vi "test_FPGAWrapper_FrameScan.vi"() -> ()   [LabVIEW 2010, in "FPGAWrapperMH120124FrameScan_PXI7813R.lvclass"]
uses:
  FPGAWrapperMH120124FrameScan_PXI7813R.lvclass
  common_typedefs/channels_cluster.ctl
  common/classes/ErrorController/ErrorController/ErrorController.lvclass
  common/classes/ErrorController/ErrorController/class_data.vi
panel:
  in  "zoom":dbl(slide)=1.0 scale=1.0..20.0
  in  "resolution":i32=256
  in  "amplitude in":dbl=3400.0
  out "FPGAWrapperMH120124FrameScan":refnum<class "FPGAWrapperMH120124FrameScan_PXI7813R.lvclass">
  out "error controller loaded?":bool=TRUE
  in  "number of channels":i32=3
  in  "block size":i32=10000
  out "channel data block":dbl[][](graph)
  in  "timeout (ms)":i32=500
  out "timed out?":bool
  out "samples read":i32
  out "DAQ loop counter":i32
  in  "iterations per pixel":i32=250
  out "pixel dwell time":dbl[unit]
  in  "channel offsets":T1
  in  "number of pixels":i32=1000000000
  in  "run button":bool
  in  "create button":bool
  in  "stop":bool
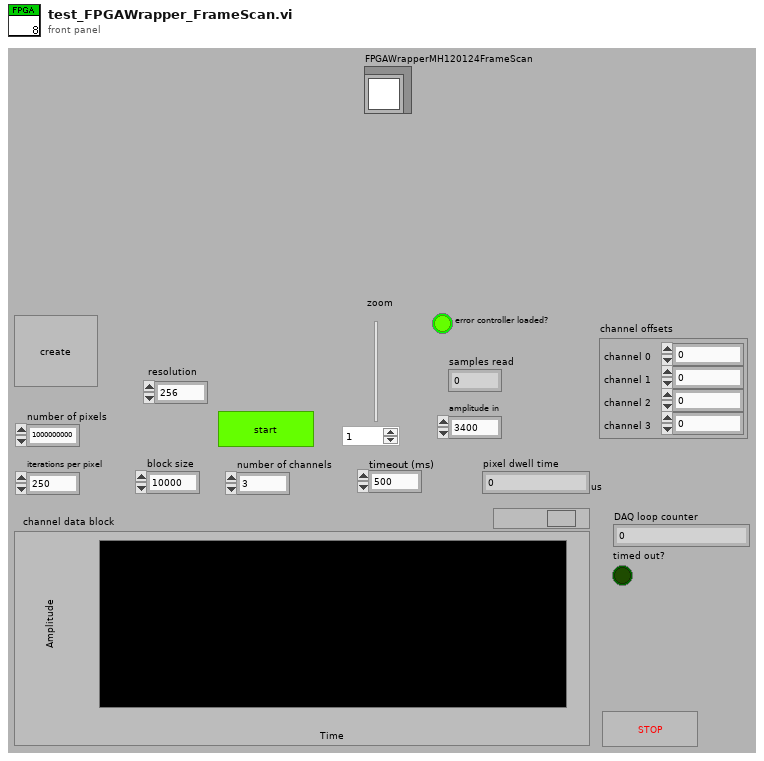
[diagram p1: front panel]
types:
  T1 = typedef "channels_cluster.ctl" = cluster{"channel 0":u32, "channel 1":u32, "channel 2":u32, "channel 3":u32}
  T2 = typedef "plugin_specification.ctl" = cluster{"class path":string, "configuration":string, "label":string, "settings name":string}
  T3 = typedef "XComponentSpecification.xctl/data.ctl" = cluster{"class path":string, "configuration":string, "label":string, "settings name":string}
  T4 = typedef "pixel_raw_data_array.ctl" = dbl[][]
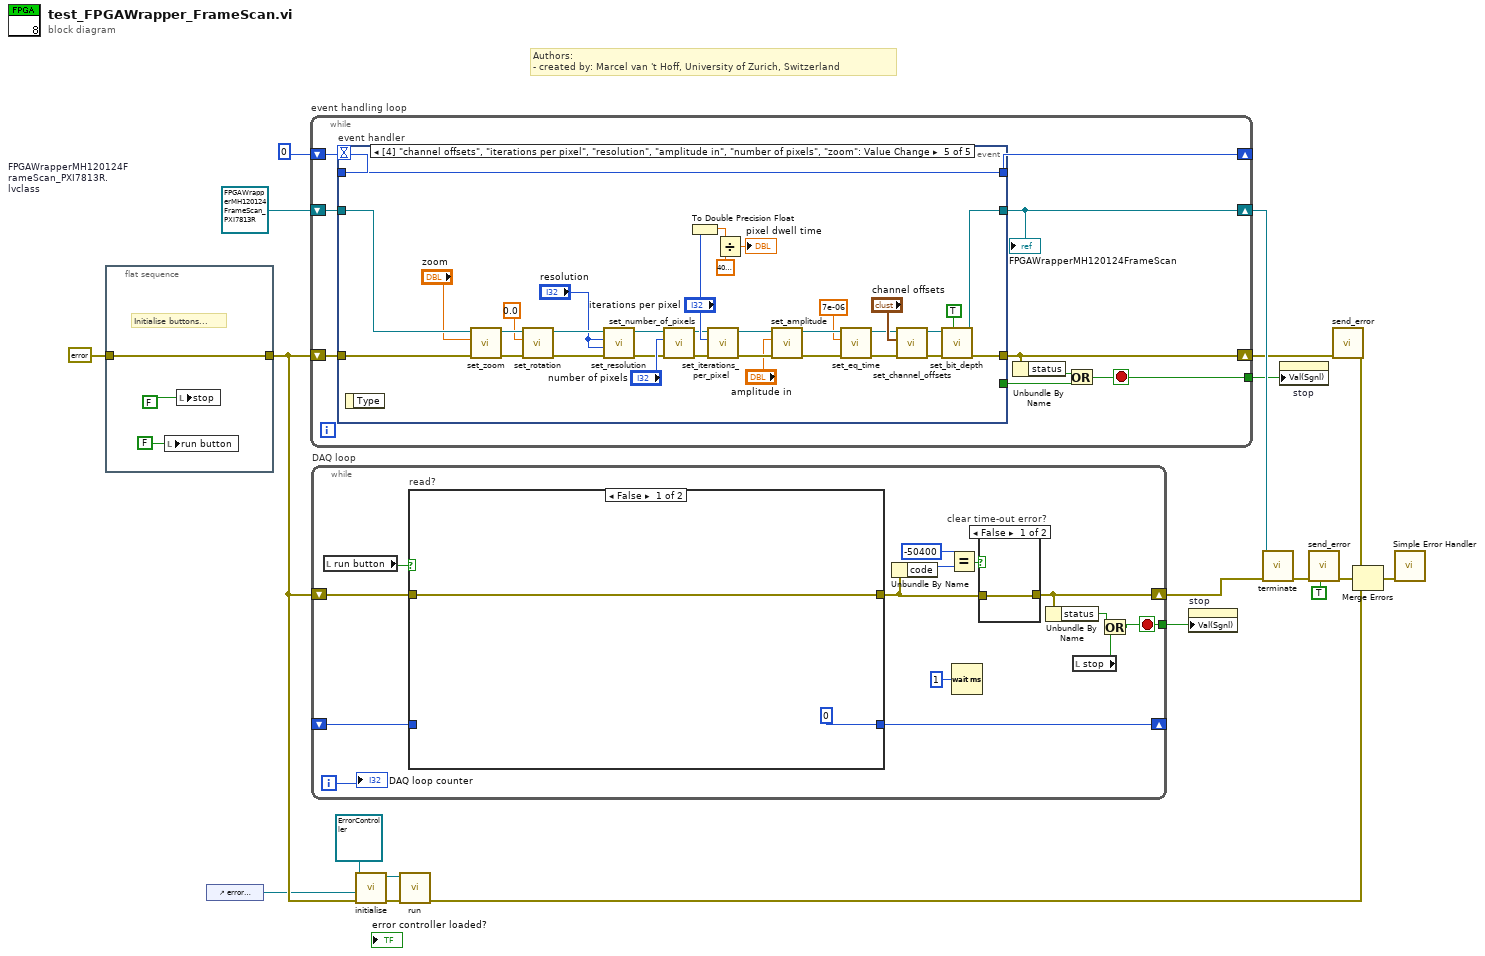
[diagram p0: block diagram]
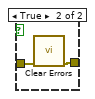
[diagram p2: hidden frame]
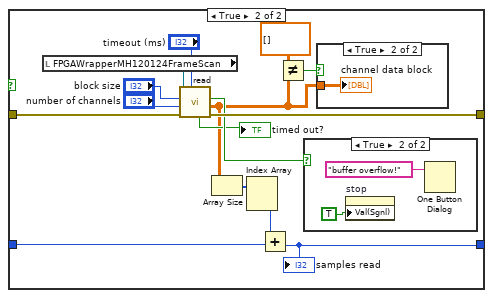
[diagram p3: hidden frame]
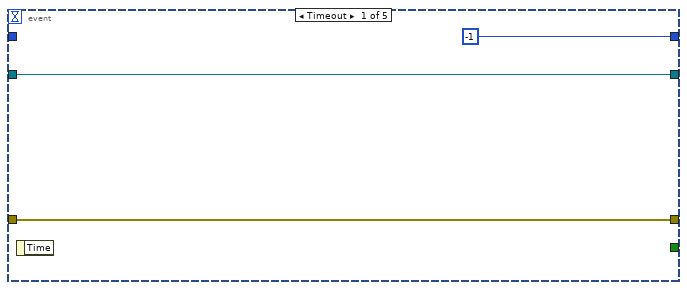
[diagram p6: hidden frame]
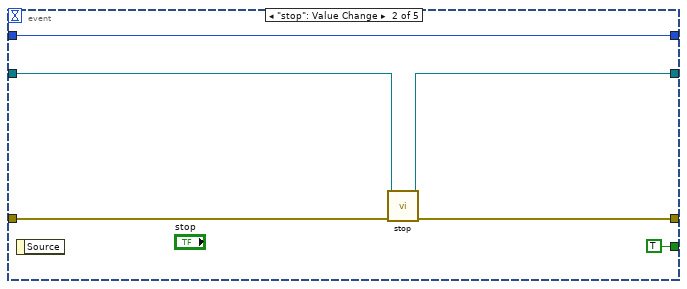
[diagram p7: hidden frame]
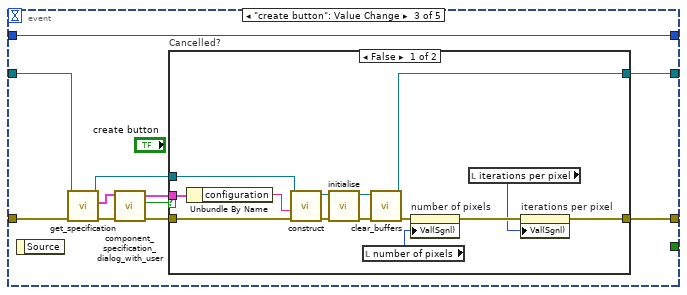
[diagram p8: hidden frame]
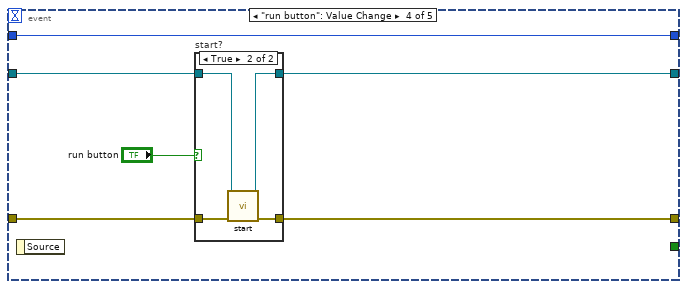
[diagram p10: hidden frame]
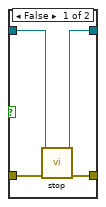
[diagram p11: hidden frame]
diagram:
  w5 = refnum<class "FPGAWrapperMH120124FrameScan_PXI7813R.lvclass"> refnum  # FPGAWrapperMH120124FrameScan_PXI7813R.lvclass
  # "Authors: \n- created by: Marcel van 't Hoff, University of Zurich, Switzerland"
  n1 = flat-sequence {
    tunnel: errorcluster {"status"=FALSE, "code"=0, "source"=""} ("error in (no error)") -> [w20]
    tunnel: [w20] -> w11
    frame #0 {
      # "Initialise buttons..."
      n2 = local write "run button"(FALSE ("run button")) -> ()
      n3 = local write "stop"(FALSE) -> ()
    }
  }
  n4 = control-ref of="error controller loaded?"() -> (w6:refnum<vi>)
  n5 = while "event handling loop" {
    shift-right: [w26] -> w2
    shift-left: w11 -> [w31]
    shift-right: [w29] -> _
    shift-left: 0 -> [w30]
    shift-right: [w27] -> w16
    shift-left: w5 -> [w28]
    tunnel: [w23] -> w3
    stop <- w23 stop-if-true
    n6 = event "event handler" shown="[4] \"channel offsets\", \"iterations per pixel\", \"resolution\", \"amplitude in\", \"number of pixels\", \"zoom\": Value Change" {
      selector: _ -> [_ _ _ _ _]
      dyn-events: _ -> [_ _ _ _ _]
      timeout: w30 -> [_ _ _ _ _]
      tunnel: [w32 w37 w50 w69 w91] -> w26
      tunnel: w31 -> [w32 w38 w47 w72 w84]
      tunnel: w30 -> [_ w40 w51 w73 w114]
      tunnel: [-1 w40 w51 w73 w114] -> w29
      tunnel: [_ TRUE _ _ _] -> w24
      tunnel: [w33 w35 w42 w70 w92] -> w27
      tunnel: w28 -> [w33 w36 w45 w71 w83]
      event Timeout {
        n7 = event-data() -> ()  [unwired: 2 out]
      }
      event "stop": Value Change {
        n8 = event-data() -> ()  [unwired: 2 out]
        n9 = call-dynamic "stop.vi"("error in (no error)"=w38, "FPGAWrapperMH120124FrameScan_PXI7813R in"=w36) -> ("error out"=w37:errorcluster, "FPGAWrapperMH120124FrameScan_PXI7813R out"=w35:refnum<class "FPGAWrapperMH120124FrameScan_PXI7813R.lvclass">)  [unwired: 8 out]
      }
      event "create button": Value Change {
        n10 = event-data() -> ()  [unwired: 2 out]
        n11 = call-dynamic "get_specification.vi"("error in (no error)"=w47, "GenericPlugin in"=w45) -> ("error out"=w46:errorcluster, "component specification"=w43:T2, "GenericPlugin out"=w44:refnum<class "FPGAWrapperMH120124FrameScan_PXI7813R.lvclass">)  [unwired: 6 in, 1 out]
        n12 = call "component_specification_dialog_with_user.vi"("error in (no error)"=w46, "component specification in"=w43) -> ("error out"=w49:errorcluster, "cancelled?"=w41:bool, "component specification out"=w48:T3)  [unwired: 7 in]
        n13 = case "Cancelled?" shown="False" w41 {
          tunnel: [w62 w67] -> w50
          tunnel: w49 -> [w56 w67]
          tunnel: w48 -> [w55 _]
          tunnel: w44 -> [w53 w66]
          tunnel: [w52 w66] -> w42
          frame False {
            n14 = Unbundle By Name(w55) -> ("configuration"=w54:string)
            n15 = call-dynamic "construct.vi"("error in (no error)"=w56, "configuration name"=w54, "GenericPlugin in"=w53) -> ("error out"=w58:errorcluster, "GenericPlugin out"=w57:refnum<class "FPGAWrapperMH120124FrameScan_PXI7813R.lvclass">)  [unwired: 7 in]
            n16 = call-dynamic "initialise.vi"("error in (no error)"=w58, "GenericPlugin in"=w57) -> ("error out"=w61:errorcluster, "GenericPlugin out"=w59:refnum<class "FPGAWrapperMH120124FrameScan_PXI7813R.lvclass">)  [unwired: 1 in, 7 out]
            n17 = local read "number of pixels"() -> (w63:i32)
            n18 = call-dynamic "clear_buffers.vi"("error in (no error)"=w61, "FPGAWrapperMH120124FrameScan_PXI7813R in"=w59) -> ("error out"=w60:errorcluster, "FPGAWrapperMH120124FrameScan_PXI7813R out"=w52:refnum<class "FPGAWrapperMH120124FrameScan_PXI7813R.lvclass">)  [unwired: 8 in]
            n19 = property on="number of pixels" class="DigNum (strict)"(error in=w60, "Val(Sgnl)"=w63) -> (error out=w65:errorcluster)  [unwired: 1 in, 1 out]
            n20 = local read "iterations per pixel"() -> (w64:i32)
            n21 = property on="iterations per pixel" class="DigNum (strict)"(error in=w65, "Val(Sgnl)"=w64) -> (error out=w62:errorcluster)  [unwired: 1 in, 1 out]
          }
          frame True {
          }
        }
      }
      event "run button": Value Change {
        n22 = event-data() -> ()  [unwired: 2 out]
        n23 = case "start?" shown="True" "run button" {
          tunnel: w72 -> [w77 w81]
          tunnel: w71 -> [w75 w80]
          tunnel: [w74 w79] -> w70
          tunnel: [w76 w78] -> w69
          frame False {
            n24 = call-dynamic "stop.vi"("error in (no error)"=w77, "FPGAWrapperMH120124FrameScan_PXI7813R in"=w75) -> ("error out"=w76:errorcluster, "FPGAWrapperMH120124FrameScan_PXI7813R out"=w74:refnum<class "FPGAWrapperMH120124FrameScan_PXI7813R.lvclass">)  [unwired: 8 out]
          }
          frame True {
            n25 = call-dynamic "start.vi"("error in (no error)"=w81, "FPGAWrapperMH120124FrameScan_PXI7813R in"=w80) -> ("error out"=w78:errorcluster, "FPGAWrapperMH120124FrameScan_PXI7813R out"=w79:refnum<class "FPGAWrapperMH120124FrameScan_PXI7813R.lvclass">)  [unwired: 8 out]
          }
        }
      }
      event "iterations per pixel", "resolution", "amplitude in", "number of pixels", "zoom": Value Change {
        n26 = event-data() -> ()  [unwired: 2 out]
        n27 = call-dynamic "set_zoom.vi"("error in (no error)"=w84, "zoom"="zoom", "FPGAWrapperMH120124FrameScan_PXI7813R in"=w83) -> ("error out"=w101:errorcluster, "FPGAWrapperMH120124FrameScan_PXI7813R out"=w102:refnum<class "FPGAWrapperMH120124FrameScan_PXI7813R.lvclass">)  [unwired: 7 in]
        n28 = call-dynamic "set_rotation.vi"("error in (no error)"=w101, "z angle (rotation angle, phi)"=dbl[unit] 0.0, "FPGAWrapperMH120124FrameScan_PXI7813R in"=w102) -> ("error out"=w99:errorcluster, "FPGAWrapperMH120124FrameScan_PXI7813R out"=w97:refnum<class "FPGAWrapperMH120124FrameScan_PXI7813R.lvclass">)  [unwired: 7 in]
        n29 = call-dynamic "set_resolution.vi"("error in (no error)"=w99, "y resolution"="resolution", "x resolution"="resolution", "FPGAWrapperMH120124FrameScan_PXI7813R in"=w97) -> ("error out"=w98:errorcluster, "FPGAWrapperMH120124FrameScan_PXI7813R out"=w96:refnum<class "FPGAWrapperMH120124FrameScan_PXI7813R.lvclass">)  [unwired: 6 in]
        n30 = call-dynamic "set_number_of_pixels.vi"("error in (no error)"=w98, "number of pixels"="number of pixels", "FPGAWrapperMH120124FrameScan_PXI7813R in"=w96) -> ("error out"=w106:errorcluster, "FPGAWrapperMH120124FrameScan_PXI7813R out"=w107:refnum<class "FPGAWrapperMH120124FrameScan_PXI7813R.lvclass">)  [unwired: 7 out]
        n31 = To Double Precision Float(number="iterations per pixel") -> (double precision float=w112:dbl)
        n32 = call-dynamic "set_iterations_per_pixel.vi"("error in (no error)"=w106, "iterations per pixel"="iterations per pixel", "FPGAWrapperMH120124FrameScan_PXI7813R in"=w107) -> ("error out"=w105:errorcluster, "FPGAWrapperMH120124FrameScan_PXI7813R out"=w104:refnum<class "FPGAWrapperMH120124FrameScan_PXI7813R.lvclass">)  [unwired: 7 out]
        n33 = Divide(x=w112, y=dbl[unit] 40000000.0) -> (x/y=→"pixel dwell time":dbl[unit])
        n34 = call-dynamic "set_amplitude.vi"("error in (no error)"=w105, "amplitude in"="amplitude in", "FPGAWrapperMH120124FrameScan_PXI7813R in"=w104) -> ("error out"=w87:errorcluster, "FPGAWrapperMH120124FrameScan_PXI7813R out"=w89:refnum<class "FPGAWrapperMH120124FrameScan_PXI7813R.lvclass">)  [unwired: 7 in]
        n35 = call-dynamic "set_eq_time.vi"("error in (no error)"=w87, "AOD equilibration time"=dbl[unit] 7e-06, "FPGAWrapperMH120124FrameScan_PXI7813R in"=w89) -> ("error out"=w86:errorcluster, "FPGAWrapperMH120124FrameScan_PXI7813R out"=w88:refnum<class "FPGAWrapperMH120124FrameScan_PXI7813R.lvclass">)  [unwired: 7 in]
        n36 = call-dynamic "set_channel_offsets.vi"("error in (no error)"=w86, "pixel values cluster"="channel offsets", "FPGAWrapperMH120124FrameScan_PXI7813R in"=w88) -> ("error out"=w93:errorcluster, "FPGAWrapperMH120124FrameScan_PXI7813R out"=w94:refnum<class "FPGAWrapperMH120124FrameScan_PXI7813R.lvclass">)  [unwired: 7 in]
        n37 = call-dynamic "set_bit_depth.vi"("calculate by timing? (F)"=TRUE, "error in (no error)"=w93, "FPGAWrapperMH120124FrameScan_PXI7813R in"=w94) -> ("error out"=w91:errorcluster, "FPGAWrapperMH120124FrameScan_PXI7813R out"=w92:refnum<class "FPGAWrapperMH120124FrameScan_PXI7813R.lvclass">)  [unwired: 7 in]
      }
    }
    "FPGAWrapperMH120124FrameScan" <- w27
    n38 = Unbundle By Name(w26) -> ("status"=w25:bool)
    n39 = Or(x=w25, y=w24) -> (x .or. y?=w23:bool)
  }
  n40 = while "DAQ loop" {
    shift-right: [w122] -> w17
    shift-left: w11 -> [w128]
    shift-right: [w117] -> _
    shift-left: _ -> [w118]
    tunnel: [w116] -> w4
    i -> [w119]
    stop <- w116 stop-if-true
    n41 = local read "run button"() -> (w127:bool)
    n42 = case "read?" shown="False" w127 {
      tunnel: w128 -> [w133 w148]
      tunnel: [w133 w147] -> w124
      tunnel: w118 -> [_ w138]
      tunnel: [0 w135] -> w117
      frame False {
      }
      frame True {
        n43 = local read "FPGAWrapperMH120124FrameScan"() -> (w146:refnum<class "FPGAWrapperMH120124FrameScan_PXI7813R.lvclass">)
        n44 = call-dynamic "read.vi"("timeout (ms)"="timeout (ms)", "error in (no error)"=w148, "number of channels"="number of channels", "block size"="block size", "FPGAWrapperMH120124FrameScan_PXI7813R in"=w146) -> ("error out"=w147:errorcluster, "channels raw data block"=w137:T4, "FIFO full?"=w141:bool, "timed out?"=→"timed out?":bool)  [unwired: 3 out]
        n45 = Array Size(array=w137) -> (size(s)=w136:i32[])
        n46 = Index Array(array=w136) -> (element #2=w134:i32)  [unwired: 2 in, 1 out]
        n47 = Add(x=w134, y=w138) -> (x+y=w135:i32)
        "samples read" <- w135
        n48 = Not Equal?(x=dbl[][] [], y=w137) -> (x != y?=w143:bool)
        n49 = case shown="True" w141 {
          frame False {
          }
          frame True {
            n50 = property on="stop" class="Bool (strict)"("Val(Sgnl)"=TRUE) -> ()  [unwired: 2 in, 2 out]
            n51 = One Button Dialog(message="buffer overflow!") -> ()  [unwired: 1 in, 1 out]
          }
        }
        n52 = case shown="True" w143 {
          tunnel: w137 -> [_ w151]
          frame False {
          }
          frame True {
            "channel data block" <- w151
          }
        }
      }
    }
    n53 = Unbundle By Name(w124) -> ("code"=w126:i32)
    n54 = Equal?(x=-50400, y=w126) -> (x = y?=w123:bool)
    n55 = Wait (ms)(milliseconds to wait=u32 1) -> ()  [unwired: 1 out]
    n56 = case "clear time-out error?" shown="False" w123 {
      tunnel: w124 -> [w129 w131]
      tunnel: [w129 w130] -> w122
      frame False {
      }
      frame True {
        n57 = call <vilib>:"Clear Errors.vi"("error in (no error)"=w131) -> ("error out"=w130:errorcluster)  [unwired: 6 out]
      }
    }
    n58 = Unbundle By Name(w122) -> ("status"=w121:bool)
    n59 = local read "stop"() -> (w120:bool)
    n60 = Or(x=w121, y=w120) -> (x .or. y?=w116:bool)
    "DAQ loop counter" <- w119
  }
  n61 = call-dynamic "initialise.vi"("error in (no error)"=w11, "error boolean"=w6, "ErrorController in"=refnum<class "ErrorController.lvclass"> refnum) -> ("error out"=w14:errorcluster, "ErrorController out"=w13:refnum<class "ErrorController.lvclass">)  [unwired: 7 in]
  n62 = call "run.vi"("error in (no error)"=w14, "ErrorController in"=w13) -> ("error out"=w7:errorcluster)  [unwired: 8 in, 1 out]
  n63 = property on="stop" class="Bool (strict)"("Val(Sgnl)"=w4) -> ()  [unwired: 2 in, 2 out]
  n64 = call-dynamic "terminate.vi"("error in (no error)"=w17, "GenericPlugin in"=w16) -> ("error out"=w10:errorcluster)  [unwired: 9 out]
  n65 = property on="stop" class="Bool (strict)"("Val(Sgnl)"=w3) -> ()  [unwired: 2 in, 2 out]
  n66 = call "send_error.vi"("last error? (F)"=TRUE, "error in (no error)"=w10) -> ("error out"=w9:errorcluster)  [unwired: 9 in]
  n67 = call "send_error.vi"("error in (no error)"=w2) -> ("error out"=w1:errorcluster)  [unwired: 10 in]
  n68 = Merge Errors(w1, w9, w7) -> (w15:errorcluster)
  n69 = call <vilib>:"Simple Error Handler.vi"("error in (no error)"=w15) -> ()  [unwired: 1 in, 8 out]
